vi "Set Strain.vi"(6 "Channel":i32=1 min=1 max=2, 8 "error in (no error)":errorcluster, 9 "Slew (V/s)":dbl, 10 "Strain (V)":dbl, 11 "RP100 in":refnum<class "RP100.lvclass">) -> (0 "error out":errorcluster, 3 "RP100 out":refnum<class "RP100.lvclass">)   [LabVIEW 2016, in "RP100.lvclass"]
doc: "Set the output <b>Strain</b> with <b>Slew</b> such that Channel 1 = -Channel 2. \n\n<b>Output Channel</b> is not used."
uses:
  RP100.lvclass
  C:/Program Files (x86)/National Instruments/LabVIEW 2016/user.lib/LevyLab/Levylab Instruments/SMOs/Instrument/Instrument.lvclass
  Typedefs/SetStrain--Cluster.ctl
  Typedefs/Commands--Enum.ctl
  <userlib>/LevyLab/Levylab Instruments/SMOs/Instrument/Instrument.lvclass
panel:
  # "legacy (not used)"
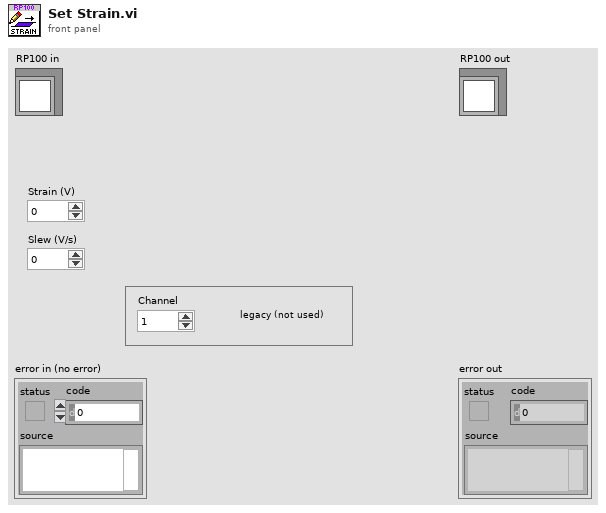
[diagram p1: front panel]
types:
  T1 = typedef "RP100.lvclass/Commands--Enum.ctl" = enum16{"setStrain", "getStrain", "setLevel", "getLevel"}
  T2 = typedef "RP100.lvclass/SetStrain--Cluster.ctl" = cluster{"Strain (V)":dbl, "Slew (V/s)":dbl}
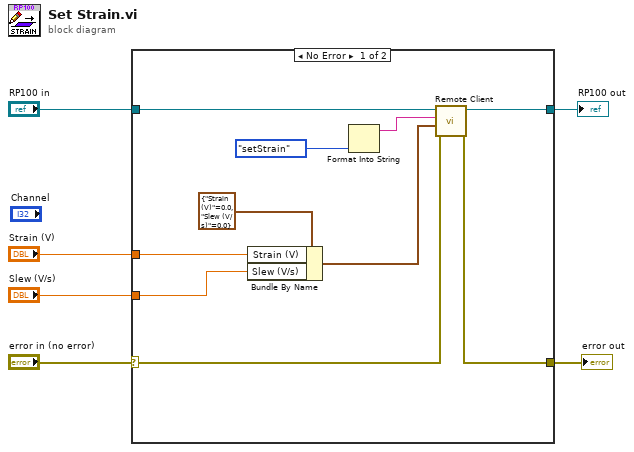
[diagram p0: block diagram]
diagram:
  n1 = case shown="No Error" "error in (no error)" {
    selector: "error in (no error)" -> [w10 w18]
    tunnel: [w9 w18] -> w5
    tunnel: "Strain (V)" -> [w15 _]
    tunnel: "RP100 in" -> [w12 w17]
    tunnel: [w11 w17] -> w2
    tunnel: "Slew (V/s)" -> [w14 _]
    frame No Error {
      n2 = Bundle By Name(cluster=T2 {"Strain (V)"=0.0, "Slew (V/s)"=0.0} ("Cluster"), "Strain (V)"=w15, "Slew (V/s)"=w14) -> (w8:T2)
      n3 = Format Into String(Commands--Enum."setStrain" ("Commands")) -> (resulting string=w13:string)  [unwired: 3 in, 1 out]
      n4 = call <userlib>:"Remote Client.vi"("error in (no error)"=w10, "Data"=w8, "Command"=w13, "Instrument in"=w12) -> ("error out"=w9:errorcluster, "Instrument out"=w11:refnum<class "RP100.lvclass">)  [unwired: 4 in, 2 out]
    }
    frame Error {
    }
  }
  "error out" <- w5
  "RP100 out" <- w2
